vi "lab2_2.vi"() -> ()   [LabVIEW 2017]
panel:
  in  "Target 2":dbl
  out "Numeric":dbl
  out "time(ms)":dbl
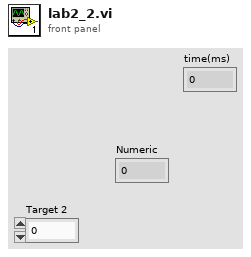
[diagram p1: front panel]
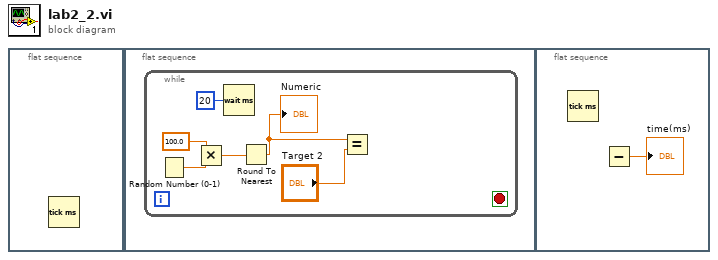
[diagram p0: block diagram]
diagram:
  n1 = flat-sequence {
    frame #0 {
      n2 = Tick Count (ms)() -> ()  [unwired: 1 out]
    }
  }
  n3 = flat-sequence {
    frame #0 {
      n4 = while {
        stop <- _ stop-if-true
        n5 = Random Number (0-1)() -> (number: 0 to 1=w5:dbl)
        n6 = Multiply(x=w5, y=100.0) -> (x*y=w3:dbl)
        n7 = Wait (ms)(milliseconds to wait=u32 20) -> ()  [unwired: 1 out]
        n8 = Round To Nearest(number=w3) -> (nearest integer value=w2:dbl)
        "Numeric" <- w2
        n9 = Equal?(x=w2, y="Target 2") -> ()  [unwired: 1 out]
      }
    }
  }
  n10 = flat-sequence {
    frame #0 {
      n11 = Tick Count (ms)() -> ()  [unwired: 1 out]
      n12 = Subtract() -> (x-y=→"time(ms)":dbl)  [unwired: 2 in]
    }
  }
